vi "Script Flatten VI.vi"(4 "Message Paths":T5, 6 "Message":T1, 7 "App":refnum<vi>, 8 "error in (no error)":errorcluster, 11 "LV-Protoc in":refnum<class "LV-Protoc.lvclass">) -> (0 "error out":errorcluster, 3 "LV-Protoc out":refnum<class "LV-Protoc.lvclass">)   [LabVIEW 2020, in "LV-Protoc.lvlib" / "LV-Protoc.lvclass"]
uses:
  LV-Protoc.lvclass
  Message Paths.ctl
  LV-Proto/Message.ctl
  LV-Proto/Field.ctl
  LV-Proto/Type.ctl
  LV-Proto/Proto Type.ctl
  LV-Protoc.lvlib
  LV-Proto/LV-Proto.lvlib
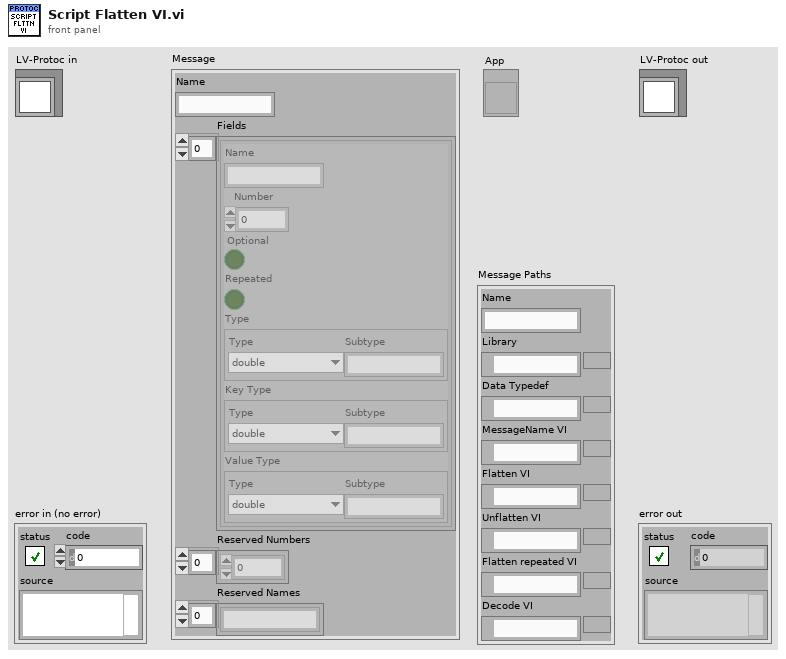
[diagram p1: front panel]
types:
  T1 = typedef "LV-Proto.lvlib/Message.ctl" = cluster{"Name":string, "Fields":T2[], "Reserved Numbers":u32[], "Reserved Names":string[]}
  T2 = typedef "LV-Proto.lvlib/Field.ctl" = cluster{"Name":string, "Number":u32, "Optional":bool, "Repeated":bool, "Type":T3, "Key Type":T3, "Value Type":T3}
  T3 = typedef "LV-Proto.lvlib/Type.ctl" = cluster{"Type":T4, "Subtype":string}
  T4 = typedef "LV-Proto.lvlib/Proto Type.ctl" = enum16{"UNKNOWN", "double", "float", "int32", "int64", "uint32", "uint64", "sint32", "sint64", "fixed32", "fixed64", "sfixed32", "sfixed64", "bool", "string", "bytes", "enum", "map", "message"}
  T5 = typedef "LV-Protoc.lvlib/Message Paths.ctl" = cluster{"Name":string, "Library":path, "Data Typedef":path, "MessageName VI":path, "Flatten VI":path, "Unflatten VI":path, "Flatten repeated VI":path, "Decode VI":path}
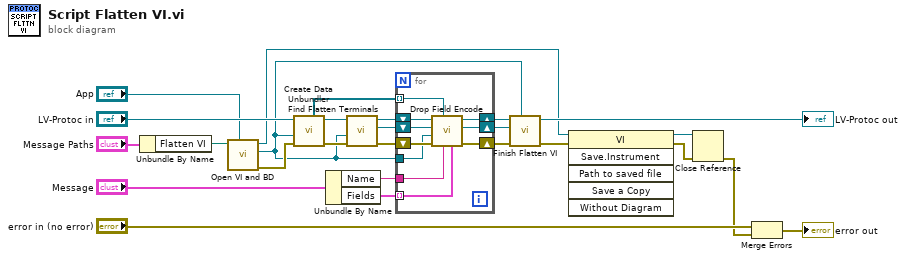
[diagram p0: block diagram]
diagram:
  n1 = Unbundle By Name("Message Paths") -> ("Flatten VI"=w4:path)
  n2 = call "Open VI and BD.vi"("App"="App", "VI Path"=w4) -> ("error out"=w26:errorcluster, "BD"=w2:refnum<vi>, "VI"=w3:refnum<vi>)  [unwired: 7 in]
  n3 = call "Create Data Unbundler.vi"("error in (no error)"=w26, "BD"=w2, "LV-Protoc in"="LV-Protoc in") -> ("error out"=w16:errorcluster, "LV-Protoc out"=w14:refnum<class "LV-Protoc.lvclass">, "Output Terminals[]"=w13:refnum<vi>[])  [unwired: 6 in]
  n4 = Unbundle By Name("Message") -> ("Name"=w21:string, "Fields"=w20:T2[])
  n5 = call "Find Flatten Terminals.vi"("error in (no error)"=w16, "BD"=w2, "LV-Protoc in"=w14) -> ("error out"=w18:errorcluster, "Output Term"=w17:refnum<vi>, "LV-Protoc out"=w19:refnum<class "LV-Protoc.lvclass">)  [unwired: 6 in]
  n6 = for {
    tunnel: w21 -> [w33]
    tunnel: w20 -> [w32] mode=indexing
    shift-right: [w30] -> w11
    shift-left: w18 -> [w36]
    shift-right: [w29] -> w9
    shift-left: w19 -> [w35]
    tunnel: w2 -> [w34]
    shift-right: [w28] -> w7
    shift-left: w17 -> [w31]
    tunnel: w13 -> [w27] mode=indexing
    n7 = call "Drop Field Encode.vi"("Field"=w32, "Message Name"=w33, "Value Terminal"=w27, "error in (no error)"=w36, "BD"=w34, "Prev Term"=w31, "LV-Protoc in"=w35) -> ("error out"=w30:errorcluster, "Output Term"=w28:refnum<vi>, "LV-Protoc out"=w29:refnum<class "LV-Protoc.lvclass">)  [unwired: 2 in]
  }
  n8 = call "Finish Flatten VI.vi"("BD"=w2, "error in (no error)"=w11, "Prev Term"=w7, "LV-Protoc in"=w9) -> ("error out"=w10:errorcluster, "LV-Protoc out"=→"LV-Protoc out":refnum<class "LV-Protoc.lvclass">)  [unwired: 6 in]
  n9 = invoke class="VI" method="Save.Instrument"(reference=w3, error in=w10) -> (reference out=w5:refnum<vi>, error out=w12:errorcluster)  [unwired: 4 in, 4 out]
  n10 = Close Reference(reference=w5, error in (no error)=w12) -> (error out=w6:errorcluster)
  n11 = Merge Errors("error in (no error)", w6) -> (→"error out":errorcluster)
